vi "S7_Init_Adapter_TCP.vi"(8 "error in":errorcluster, 10 "Timeout":u32=5000, 11 "TCP Connection Ref":refnum<k5>) -> (0 "error out":errorcluster, 2 "Connected":bool, 3 "TCP Connection Ref Out":refnum<k5>)   [LabVIEW 2018, in "S7 TCP.lvlib"]
uses:
  S7 TCP.lvlib
panel:
  in  "Slot#":u8 format="%.0x"
  out "Attempts":i32
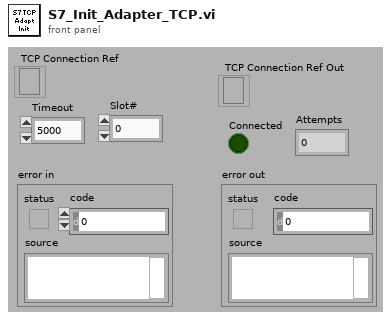
[diagram p1: front panel]
types:
  T1 = enum16{"Standard", "Buffered", "CRLF", "Immediate"}
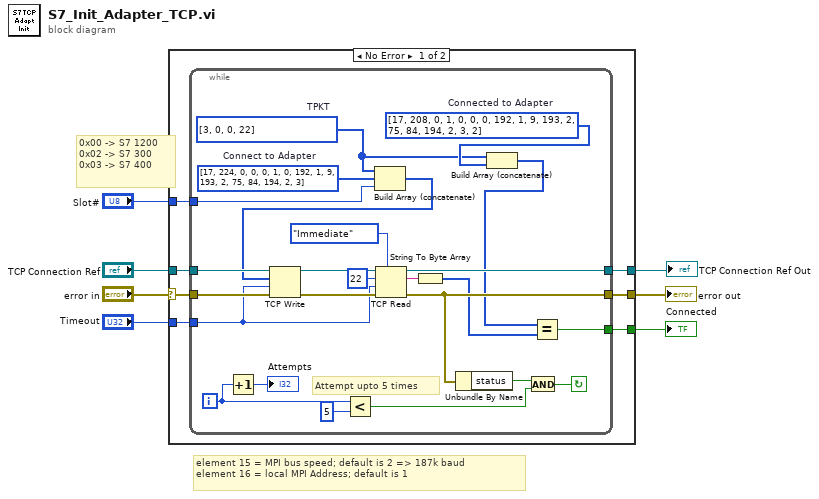
[diagram p0: block diagram]
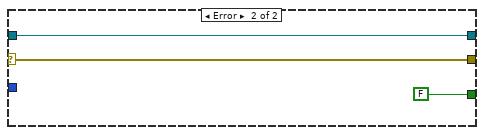
[diagram p2: hidden frame]
diagram:
  # "0x00 -> S7 1200\n0x02 -> S7 300\n0x03 -> S7 400"
  # "element 15 = MPI bus speed; default is 2 => 187k baud\nelement 16 = local MPI Address; default is 1"
  n1 = case shown="No Error" "error in" {
    selector: "error in" -> [w13 w41]
    tunnel: [w12 w40] -> w2
    tunnel: [w11 w41] -> w6
    tunnel: "TCP Connection Ref" -> [w14 w40]
    tunnel: [w10 FALSE] -> w5
    tunnel: "Timeout" -> [w9 _]
    tunnel: "Slot#" -> [w8 _]
    frame No Error {
      n2 = while {
        tunnel: w14 -> [w31]
        tunnel: w13 -> [w30]
        tunnel: [w26] -> w12
        tunnel: [w27] -> w11
        tunnel: [w38] -> w10
        tunnel: w9 -> [w24]
        tunnel: w8 -> [w15]
        i -> [w36]
        stop <- w37 continue-if-true
        w19 = u8[] [17, 208, 0, 1, 0, 0, 0, 192, 1, 9, 193, 2, 75, 84, 194, 2, 3, 2]  # Connected to Adapter
        w18 = u8[] [3, 0, 0, 22]  # TPKT
        w21 = u8[] [17, 224, 0, 0, 0, 1, 0, 192, 1, 9, 193, 2, 75, 84, 194, 2, 3]  # Connect to Adapter
        # "Attempt upto 5 times"
        n3 = Increment(x=w36) -> (x+1=→"Attempts":i32)
        n4 = Less?(x=w36, y=5) -> (x < y?=w34:bool)
        n5 = Build Array (concatenate)(w18, w21, w15) -> (w20:u8[])
        n6 = TCP Write(connection ID=w31, data in=w20, error in (no error)=w30, 9:w24) -> (connection ID out=w29:refnum<k5>, error out=w28:errorcluster)  [unwired: 1 out]
        n7 = TCP Read(connection ID=w29, bytes to read=22, error in (no error)=w28, 7:T1."Immediate" ("mode (standard)"), 9:w24) -> (connection ID out=w26:refnum<k5>, data out=w22:string, error out=w27:errorcluster)
        n8 = String To Byte Array(string=w22) -> (unsigned byte array=w17:u8[])
        n9 = Unbundle By Name(w27) -> ("status"=w32:bool)
        n10 = Build Array (concatenate)(w18, w19) -> (w16:u8[])
        n11 = And(x=w32, y=w34) -> (x .and. y?=w37:bool)
        n12 = Equal?(x=w16, y=w17) -> (x = y?=w38:bool)
      }
    }
    frame Error {
    }
  }
  "error out" <- w6
  "Connected" <- w5
  "TCP Connection Ref Out" <- w2
